vi "IPS120 WH3 - Write Setrate.vi"(0 "Setrate":dbl format="%.2f", 1 "GPIB Address":string) -> ()   [LabVIEW 2009]
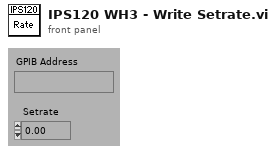
[diagram p1: front panel]
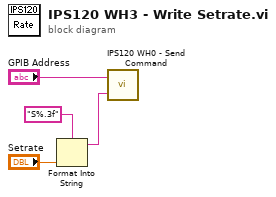
[diagram p0: block diagram]
diagram:
  n1 = Format Into String(format string="S%.3f", "Setrate") -> (resulting string=w1:string)  [unwired: 2 in, 1 out]
  n2 = call "IPS120 WH0 - Send Command.vi"("Command String"=w1, "GPIB Address"="GPIB Address") -> ()  [unwired: 1 out]
